vi "Apply_ROI_IMAQdx.vi"(8 "error in (no error)":errorcluster={"status"=TRUE, "code"=-1074360304, "source"="Property Node (arg 2) in Tail_Deflection_Fixed_Head_Basler.vi"}, 9 "Steps":T1={"OffsetX Step"=8, "Width Step"=8, "OffsetY Step"=2, "Height Step"=2}, 10 "ROI":T2={"Left"=0, "Top"=0, "Right"=639, "Bottom"=479, "Rotation"=0.0} {"Rotation" min=-90.0 max=90.0 step=1.0 format="%.2f"; "Left" scale=0.0..1024.0; "Right" scale=0.0..1024.0}, 11 "Session in":T3="cam1") -> (0 "error out":errorcluster={"status"=TRUE, "code"=-1074360304, "source"="Property Node (arg 2) in Tail_Deflection_Fixed_Head_Basler.vi"}, 1 "Size":cluster{"X":i32, "Y":i32}={"X"=640, "Y"=480}, 2 "Actual ROI":T2={"Left"=0, "Top"=0, "Right"=639, "Bottom"=479, "Rotation"=0.0} {"Rotation" format="%.2f"; "Left" scale=0.0..1024.0; "Right" scale=0.0..1024.0}, 3 "Session out":T3="cam1")   [LabVIEW 2019]
uses:
  <vilib>/userDefined/High Color/IMAQdx.ctl
  <resource>/objmgr/imaqdx.rc
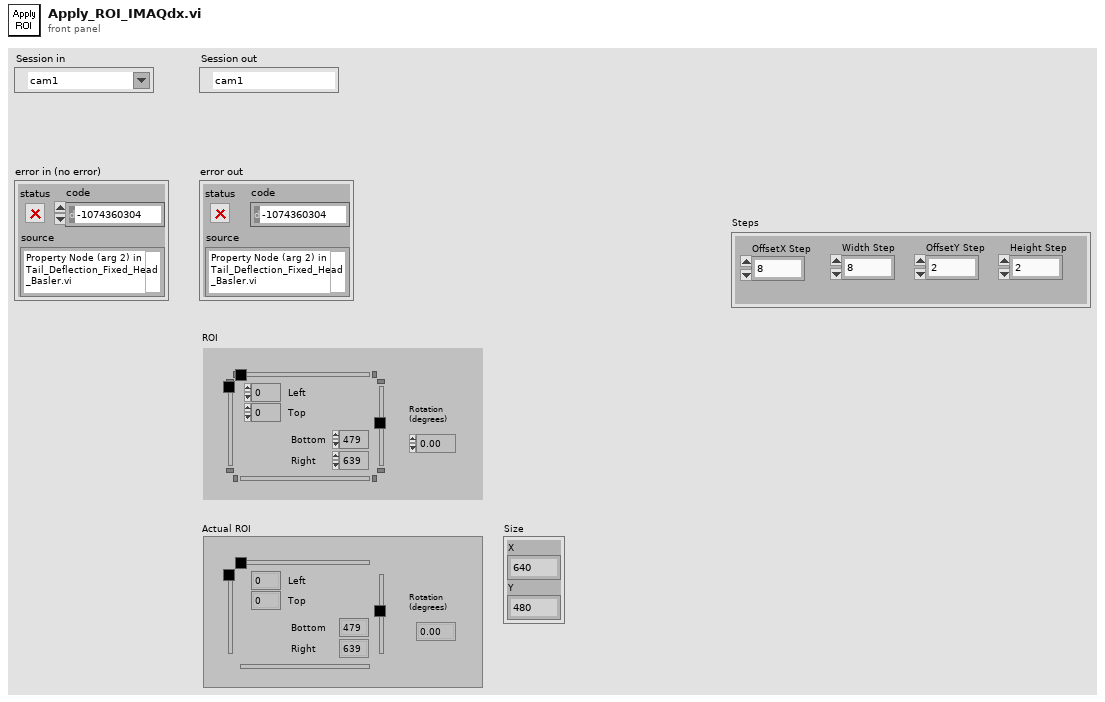
[diagram p1: front panel]
types:
  T1 = cluster{"OffsetX Step":i32, "Width Step":i32, "OffsetY Step":i32, "Height Step":i32}
  T2 = typedef "IMAQ Rectangle" = cluster{"Left":i32, "Top":i32, "Right":i32, "Bottom":i32, "Rotation":dbl}
  T3 = typedef "IMAQdx.ctl" = refnum<k21>
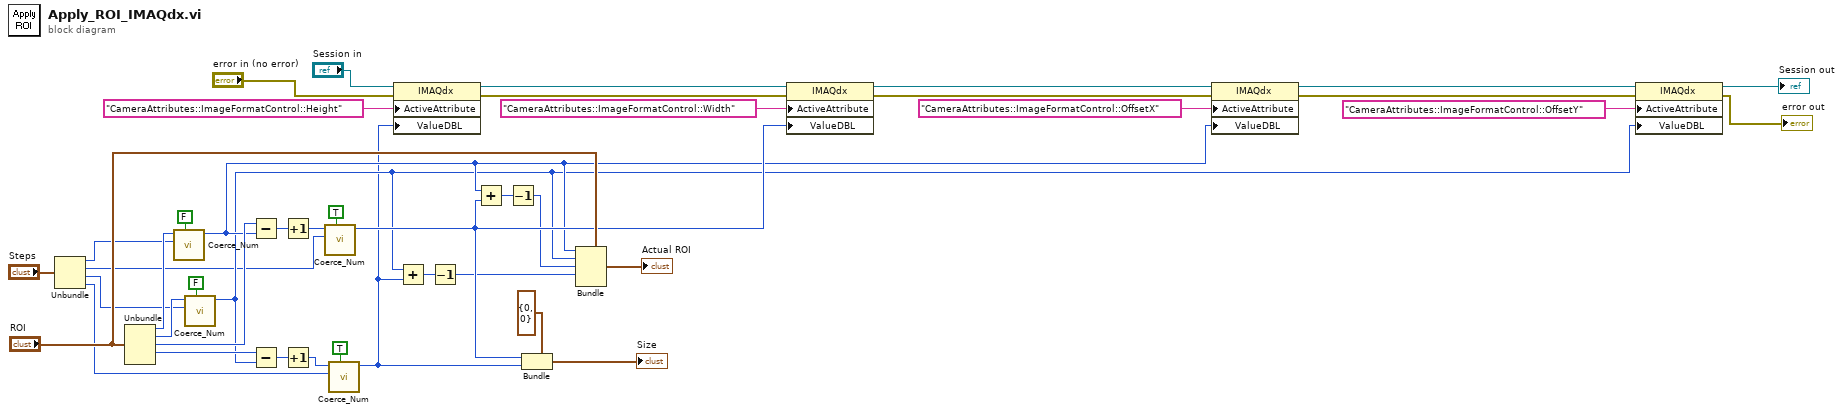
[diagram p0: block diagram]
diagram:
  n1 = Unbundle("Steps") -> ("OffsetX Step"=w5:i32, "Width Step"=w4:i32, "OffsetY Step"=w3:i32, "Height Step"=w2:i32)
  n2 = Unbundle("ROI") -> ("Left"=w20:i32, "Top"=w17:i32, "Right"=w24:i32, "Bottom"=w37:i32)  [unwired: 1 out]
  n3 = call "Coerce_Num.vi"("Coerce towards +infinite?"=FALSE, "Num Step"=w5, "Num In"=w20) -> ("Num Out"=w10:i32)  [unwired: 8 in]
  n4 = call "Coerce_Num.vi"("Coerce towards +infinite?"=FALSE, "Num Step"=w3, "Num In"=w17) -> ("Num Out"=w9:i32)  [unwired: 8 in]
  n5 = Subtract(x=w24, y=w10) -> (x-y=w36:i32)
  n6 = Subtract(x=w37, y=w9) -> (x-y=w35:i32)
  n7 = Increment(x=w36) -> (x+1=w15:i32)
  n8 = Increment(x=w35) -> (x+1=w13:i32)
  n9 = call "Coerce_Num.vi"("Coerce towards +infinite?"=TRUE, "Num Step"=w4, "Num In"=w15) -> ("Num Out"=w12:i32)  [unwired: 8 in]
  n10 = call "Coerce_Num.vi"("Coerce towards +infinite?"=TRUE, "Num Step"=w2, "Num In"=w13) -> ("Num Out"=w1:i32)  [unwired: 8 in]
  n11 = property class="IMAQdx"(reference="Session in", error in="error in (no error)", "ActiveAttribute"="CameraAttributes::ImageFormatControl::Height", "ValueDBL"=w1) -> (reference out=w39:T3, error out=w38:errorcluster)
  n12 = Add(x=w9, y=w1) -> (x+y=w11:i32)
  n13 = Decrement(x=w11) -> (x-1=w7:i32)
  n14 = Add(x=w10, y=w12) -> (x+y=w25:i32)
  n15 = Decrement(x=w25) -> (x-1=w8:i32)
  n16 = Bundle(cluster=cluster{"X":i32, "Y":i32} {"X"=0, "Y"=0} ("Start Point"), "X"=w12, "Y"=w1) -> (→"Size":cluster{"X":i32, "Y":i32})
  n17 = Bundle(cluster="ROI", "Left"=w10, "Top"=w9, "Right"=w8, "Bottom"=w7) -> (→"Actual ROI":T2)  [unwired: 1 in]
  n18 = property class="IMAQdx"(reference=w39, error in=w38, "ActiveAttribute"="CameraAttributes::ImageFormatControl::Width", "ValueDBL"=w12) -> (reference out=w32:T3, error out=w31:errorcluster)
  n19 = property class="IMAQdx"(reference=w32, error in=w31, "ActiveAttribute"="CameraAttributes::ImageFormatControl::OffsetX", "ValueDBL"=w10) -> (reference out=w30:T3, error out=w29:errorcluster)
  n20 = property class="IMAQdx"(reference=w30, error in=w29, "ActiveAttribute"="CameraAttributes::ImageFormatControl::OffsetY", "ValueDBL"=w9) -> (reference out=→"Session out":T3, error out=→"error out":errorcluster)
